vi "nonlinear_calibration_load(subVI).vi"(8 "error in (no error)":errorcluster, 9 "Grid Descriptor":cluster{"X Step":sgl, "Y Step":sgl, "Unit":T2}={"X Step"=10.0, "Y Step"=10.0, "Unit"=enum."Millimeter"}, 10 "name or relative path":path=path "calib-info.jpg", 11 "File Path":path) -> (0 "error out":errorcluster, 1 "calibration image":T1, 2 "Error Statistics":T4, 3 "Calibration Axis Info":T3={"Origin Pixel"={"X"=0.0, "Y"=0.0}, "Angle Relative to Horizontal (deg)"=0.0, "X Axis Pixel"={"X"=0.0, "Y"=0.0}, "Axis Reference"=1} {"X Axis Pixel"."Y" format="%.2f"; "X Axis Pixel"."X" format="%.2f"; "Axis Reference" items=["Direct", "Indirect"]; "Angle Relative to Horizontal (deg)" format="%.2f"; "Origin Pixel"."Y" format="%.2f"; "Origin Pixel"."X" format="%.2f"})   [LabVIEW 2020]
uses:
  <vilib>/vision/Calibration.llb/Error Statistics.ctl
  <vilib>/vision/Image Controls.llb/IMAQ Image.ctl
  <vilib>/vision/Calibration.llb/Distortion Model.ctl
  <vilib>/vision/Calibration.llb/Distortion Model Types.ctl
  <vilib>/vision/NI_Vision_Development_Module.lvlib
panel:
  out "Error Map":sgl[][](array[numeric]) format="%.2f"
  out "Image":T1(plugin-control)
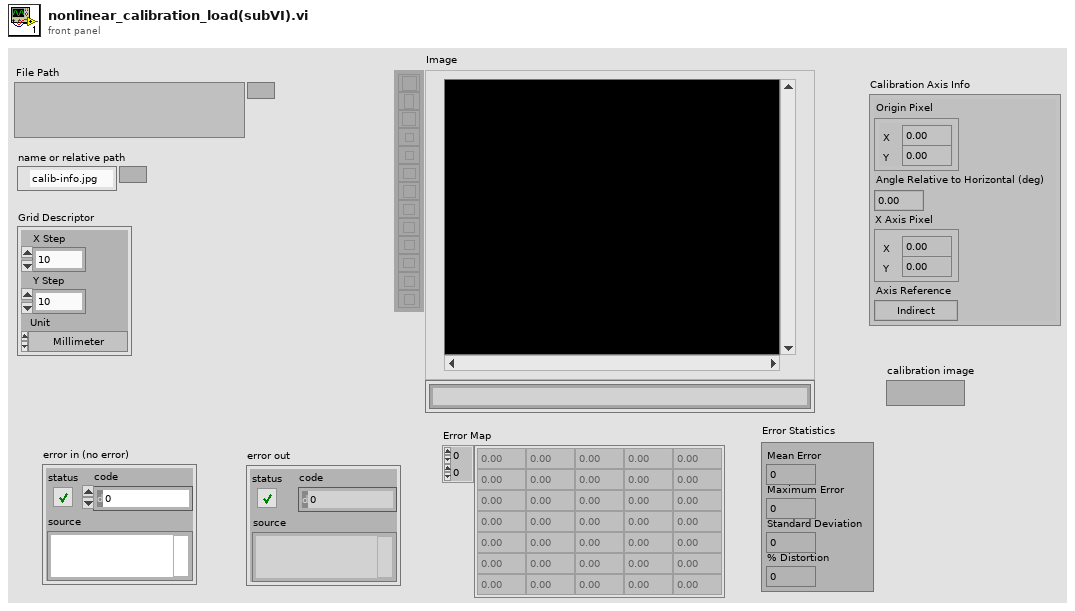
[diagram p1: front panel]
types:
  T1 = typedef "IMAQ Image.ctl" = refnum<image>
  T2 = typedef "Image Unit" = enum32{"Undefined", "Angström", "Micrometer", "Millimeter", "Centimeter", "Meter", "Kilometer", "Microinch", "Inch", "Feet", "Nautical miles", "Standard miles", "Steps"}
  T3 = cluster{"Origin Pixel":cluster{"X":sgl, "Y":sgl}, "Angle Relative to Horizontal (deg)":sgl, "X Axis Pixel":cluster{"X":sgl, "Y":sgl}, "Axis Reference":u32}
  T4 = typedef "Error Statistics.ctl" = cluster{"Mean Error":dbl, "Maximum Error":dbl, "Standard Deviation":dbl, "% Distortion":dbl}
  T5 = cluster{"Origin Pixel":cluster{"X":sgl, "Y":sgl}, "Angle Relative to Horizontal (deg)":sgl, "Axis Reference":u32}
  T6 = typedef "Distortion Model.ctl" = cluster{"Distortion Model":T7, "Polynomial Model Setup":cluster{"Radial Coefficient":u32, "Tangential Coefficients ":bool}}
  T7 = typedef "Distortion Model Types.ctl" = i32
  T8 = typedef "Particle Parameters" = i32
  T9 = cluster{"Measurement Parameter":T8, "Range Lower Value":dbl, "Range Upper Value":dbl, "Range":bool, "Measurement Type":bool}[]
  T10 = typedef "Calibration Reference Points.ctl" = cluster{"Pixel Coordinates":cluster{"X":dbl, "Y":dbl}[], "Real World Coordinates":cluster{"X":dbl, "Y":dbl}[], "Unit":T2, "Image Size":cluster{"X":u32, "Y":u32}}
  T11 = cluster{"Desired Font (Application)":enum16{"User-specified Font", "Application Font", "System Font", "Dialog Font"}, "[User-specified Font]":cluster{"Font Name":string, "Size":i16, "Strikeout?":bool, "Italic?":bool, "Underline?":bool, "Outline?":bool, "Shadow?":bool, "Bold?":bool, "Rotation Angle":dbl}, "Horizontal Alignment":i16, "Vertical Alignment":i16}
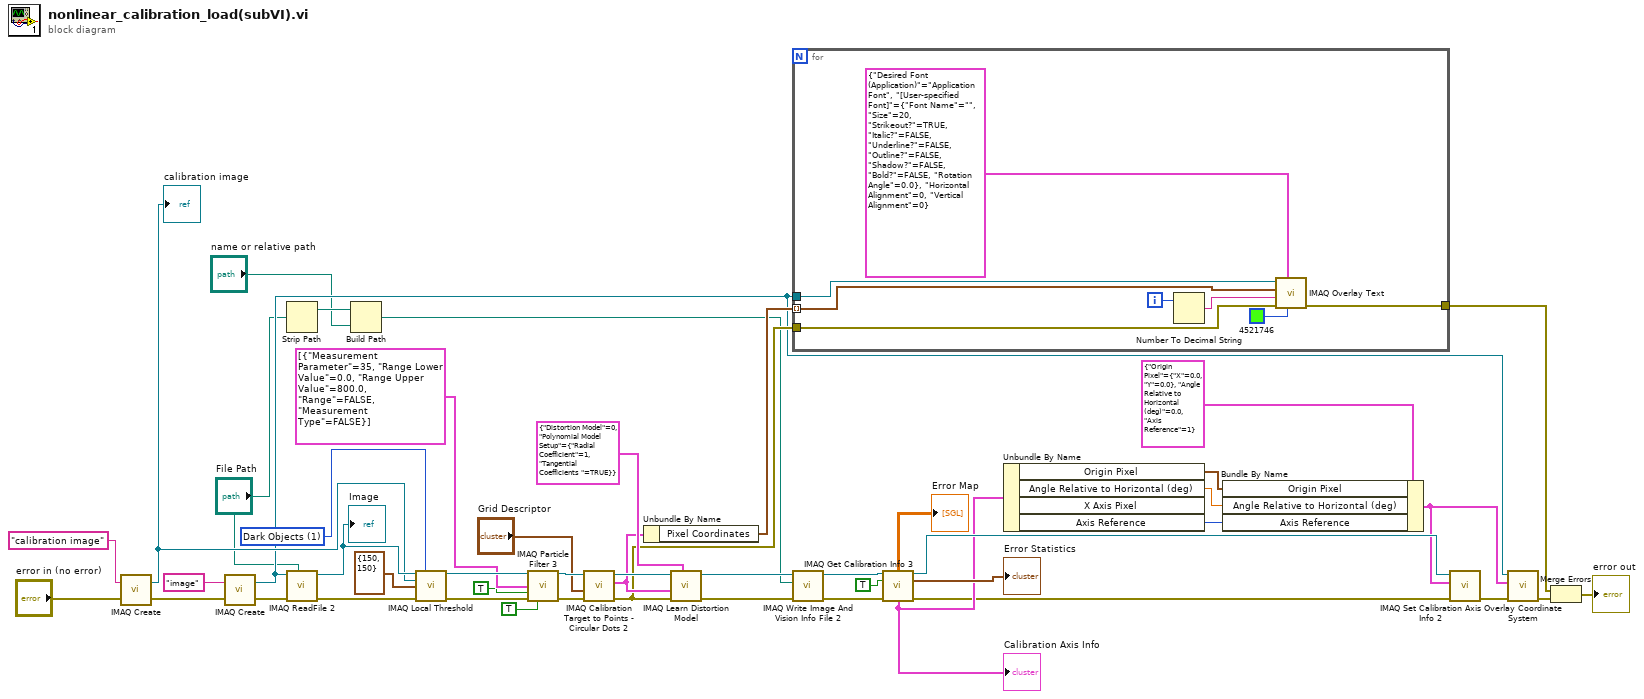
[diagram p0: block diagram]
diagram:
  w34 = u32 1 items=["Bright Objects", "Dark Objects"] ("Look For (Bright Objects)")
  n1 = call "IMAQ Create"("Image Name"="calibration image", "error in (no error)"="error in (no error)") -> ("New Image"=w23:T1, "error out"=w21:errorcluster)  [unwired: 3 in]
  "calibration image" <- w23
  n2 = call "IMAQ Create"("Image Name"="image", "error in (no error)"=w21) -> ("New Image"=w12:T1, "error out"=w44:errorcluster)  [unwired: 3 in]
  n3 = Strip Path(path="File Path") -> (stripped path=w3:path)  [unwired: 1 out]
  n4 = call "IMAQ ReadFile 2"("File Path"="File Path", "error in (no error)"=w44, "Image"=w12) -> ("error out"=w43:errorcluster, "Image Out"=w39:T1)  [unwired: 4 in, 3 out]
  "Image" <- w39
  n5 = Build Path(base path=w3, name or relative path="name or relative path") -> (appended path=w1:path)
  n6 = call "IMAQ Local Threshold"("Image Src"=w39, "Look For (Bright Objects)"=w34, "Image Dst"=w23, "Window Size (32x32)"=cluster{"SizeX":i32, "SizeY":i32} {"SizeX"=150, "SizeY"=150}, "error in (no error)"=w43) -> ("Image Dst Out"=w47:T1, "error out"=w42:errorcluster)  [unwired: 9 in]
  n7 = call "IMAQ Particle Filter 3"("Image Src"=w47, "Selection Values"=T9 [{"Measurement Parameter"=35, "Range Lower Value"=0.0, "Range Upper Value"=800.0, "Range"=FALSE, "Measurement Type"=FALSE}], "Keep/Remove Particles (F)"=TRUE, "error in (no error)"=w42, "Reject Border? (F)"=TRUE) -> ("Image Dst Out"=w45:T1, "error out"=w41:errorcluster)  [unwired: 8 in, 1 out]
  n8 = call "IMAQ Calibration Target to Points - Circular Dots 2"("error in (no error)"=w41, "Grid Descriptor"="Grid Descriptor", "Target Image"=w45) -> ("error out"=w27:errorcluster, "Reference Points"=w28:T10, "Target Image (dup)"=w46:T1)  [unwired: 6 in]
  n9 = Unbundle By Name(w28) -> ("Pixel Coordinates"=w24:cluster{"X":dbl, "Y":dbl}[])
  n10 = call "IMAQ Learn Distortion Model"("Distortion Model Setup"=T6 {"Distortion Model"=0, "Polynomial Model Setup"={"Radial Coefficient"=1, "Tangential Coefficients "=TRUE}}, "error in (no error)"=w27, "Reference Points"=w28, "Calibration Template Image"=w46) -> ("error out"=w8:errorcluster, "Calibration Template Image Out"=w6:T1)  [unwired: 6 in]
  n11 = for {
    tunnel: w12 -> [w55]
    tunnel: w27 -> [w54]
    tunnel: [w53] -> w26
    tunnel: w24 -> [w52] mode=indexing
    i -> [w51]
    n12 = Number To Decimal String(number=w51) -> (decimal integer string=w50:string)  [unwired: 1 in]
    n13 = call "IMAQ Overlay Text"("Text Color (black)"=u32 4521746, "Font, Size & Style"=T11 {"Desired Font (Application)"=enum."Application Font", "[User-specified Font]"={"Font Name"="", "Size"=20, "Strikeout?"=TRUE, "Italic?"=FALSE, "Underline?"=FALSE, "Outline?"=FALSE, "Shadow?"=FALSE, "Bold?"=FALSE, "Rotation Angle"=0.0}, "Horizontal Alignment"=0, "Vertical Alignment"=0}, "error in (no error)"=w54, "String"=w50, "Origin"=w52, "Image"=w55) -> ("error out"=w53:errorcluster)  [unwired: 4 in, 1 out]
  }
  n14 = call "IMAQ Write Image And Vision Info File 2"("error in (no error)"=w8, "File Path"=w1, "Image"=w6) -> ("error out"=w7:errorcluster, "Image Out (duplicate)"=w5:T1)  [unwired: 7 in]
  n15 = call "IMAQ Get Calibration Info 3"("Calibration Template Image"=w5, "Return Error Information (False)"=TRUE, "error in (no error)"=w7) -> ("Error Map"=→"Error Map":sgl[][], "Calibration Template Image (duplicate)"=w19:T1, "Error Statistics"=→"Error Statistics":T4, "Calibration Axis Info"=w18:T3, "error out"=w13:errorcluster)  [unwired: 4 in, 4 out]
  "Calibration Axis Info" <- w18
  n16 = Unbundle By Name(w18) -> ("Origin Pixel"=w16:cluster{"X":sgl, "Y":sgl}, "Angle Relative to Horizontal (deg)"=w15:sgl, "Axis Reference"=w14:u32)  [unwired: 1 out]
  n17 = Bundle By Name(cluster=T5 {"Origin Pixel"={"X"=0.0, "Y"=0.0}, "Angle Relative to Horizontal (deg)"=0.0, "Axis Reference"=1} ("Calibration Axis Info 2"), "Origin Pixel"=w16, "Angle Relative to Horizontal (deg)"=w15, "Axis Reference"=w14) -> (w11:T5)
  n18 = call-poly "IMAQ Set Calibration Axis Info 2"("error in (no error)"=w13, "Calibration Axis Info"=w11, "Calibration Template Image In"=w19) -> ("error out"=w10:errorcluster)  [unwired: 7 in, 1 out]
  n19 = call "Overlay Coordinate System.vi"("error in"=w10, "Calibration Axis Info"=w11, "Image"=w12) -> ("error out"=w9:errorcluster)  [unwired: 7 in, 1 out]
  n20 = Merge Errors(w26, w9) -> (→"error out":errorcluster)
